vi "helper-log-eng.vi"(8 "error in":errorcluster, 10 "ARGS":string, 11 "case":T1) -> (0 "error out":errorcluster, 3 "Collected Reports":string)   [LabVIEW 2024]
uses:
  controls/state-engine.ctl
  controls/enum.report-filter.ctl
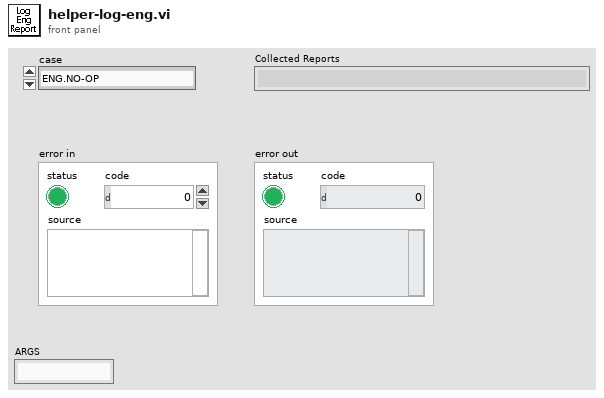
[diagram p1: front panel]
types:
  T1 = typedef "state-engine.ctl" = enum16{"ENG.NO-OP", "ENG.START", "ENG.STOP", "ENG.EXECUTE", "ENG.STATUS", "ENG.EXTERNAL-CALL", "ENG.INIT", "ENG.INIT.VARS", "ENG.INIT.SERIAL", "ENG.LOAD", "ENG.LOAD.SINGLE", "ENG.LOAD.MODULE", "ENG.LOAD.RELOAD", "ENG.LOAD.UNLOAD", "ENG.IO.LOAD", "ENG.IO.SAVE", "ENG.PROC.RELOAD-BY-NAME", "ENG.PROC.START", "ENG.PROC.STOP", "ENG.PROC.INSERT-STEPS", "ENG.PROC.ISRUNNING", "ENG.PROC.PRESET", "ENG.PROC.STATUS", "ENG.PRINT-USER-MSG", "ENG.RIO.SNAPSHOT", "ENG.RIO.AIN-SNAPSHOT-CALIB", "ENG.RIO.DOUT-BY-ADDR", "ENG.RIO.DOUT-BY-NAME", "ENG.RIO.RFS-DELAY-SET-X1", "ENG.RIO.RFS-DELAY-SET-X8", "ENG.RIO.RFS-CYCLES-SET", "ENG.RIO.RFS-CYCLES-GET", "ENG.RIO.RFS-ENABLE", "ENG.EXIT"}
  T2 = typedef "enum.report-filter.ctl" = enum16{"Read ALL", "Read Errors", "Collect", "ClearAll"}
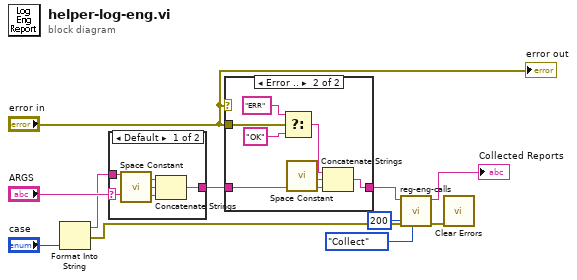
[diagram p0: block diagram]
diagram:
  n1 = Format Into String("case") -> (resulting string=w7:string, error out=w5:errorcluster)  [unwired: 3 in]
  n2 = case shown="Default" "ARGS" {
    selector: "ARGS" -> [w13 _]
    tunnel: [w12 w16] -> w4
    tunnel: w7 -> [w15 w16]
    frame Default {
      n3 = call <vilib>:"Space Constant.vi"() -> ("String"=w14:string)
      n4 = Concatenate Strings(w15, w14, w13) -> (w12:string)
    }
    frame "" {
    }
  }
  n5 = case shown="Error .." "error in" {
    tunnel: "error in" -> [_ w24]
    tunnel: w4 -> [w17 w18]
    tunnel: [w17 w22] -> w3
    frame No Error {
    }
    frame Error {
      n6 = Select(t="ERR" ("String"), s=w24, f="OK" ("String")) -> (s? t:f=w19:string)
      n7 = call <vilib>:"Space Constant.vi"() -> ("String"=w23:string)
      n8 = Concatenate Strings(w19, w23, w18) -> (w22:string)
    }
  }
  n9 = call "reg-eng-calls.vi"("Operation(Read)"=enum.report-filter."Collect", "error in"=w5, "Rows"=200, "Reports to Collect"=w3) -> ("error out"=w6:errorcluster, "Collected Reports"=→"Collected Reports":string)  [unwired: 6 in]
  n10 = call <vilib>:"Clear Errors.vi"("error in (no error)"=w6) -> ()  [unwired: 5 in, 2 out]
  "error out" <- "error in"
